vi "CC Script Parse Define.vi"(8 "error in (no error)":errorcluster, 9 "To String?":bool, 10 "Object in":T1, 11 "DefineObject Parameters":string="\"Object Name\" RA=12:32:25.123,DEC=45:22:33.234, muDEC=123.45, Epoch=12.345") -> (0 "error out":errorcluster, 1 "Name":string, 2 "Script":string, 3 "Object out":T1)   [LabVIEW 2024]
uses:
  typedefs/CC cluster Object.ctl
  typedefs/CC cluster sidereal rate.ctl
  typedefs/CC cluster RA and DEC.ctl
  typedefs/cc cluster muRA muDEC.ctl
  Telescope/CC cluster Telescope Offsets.ctl
  <vilib>/regexp/Match Regular Expression.xnode
panel:
  # "\"Object Name\" RA=HH:MM:SS.nnn,DEC=DEG:MM:SS.nnn, muDEC=nnn.nn, Epoch=nn.nnn"
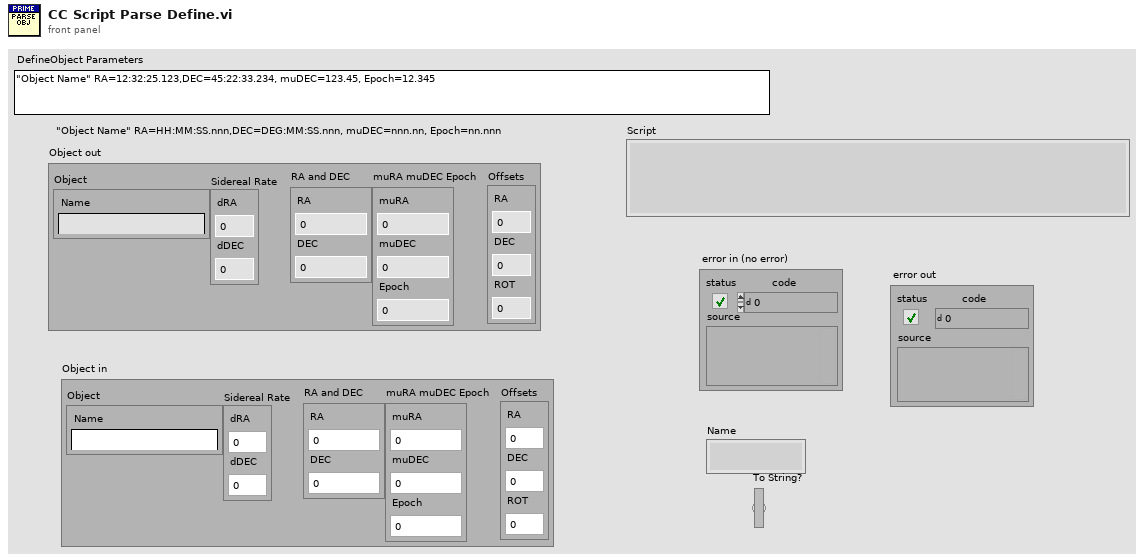
[diagram p1: front panel]
types:
  T1 = typedef "CC cluster Object.ctl" = cluster{"Object":cluster{"Name":string}, "Sidereal Rate":T2, "RA and DEC":T3, "muRA muDEC Epoch":T4, "Offsets":T5}
  T2 = typedef "CC cluster sidereal rate.ctl" = cluster{"dRA":dbl, "dDEC":dbl}
  T3 = typedef "CC cluster RA and DEC.ctl" = cluster{"RA":dbl, "DEC":dbl}
  T4 = typedef "cc cluster muRA muDEC.ctl" = cluster{"muRA":dbl, "muDEC":dbl, "Epoch":dbl}
  T5 = typedef "CC cluster Telescope Offsets.ctl" = cluster{"RA":dbl, "DEC":dbl, "ROT":dbl}
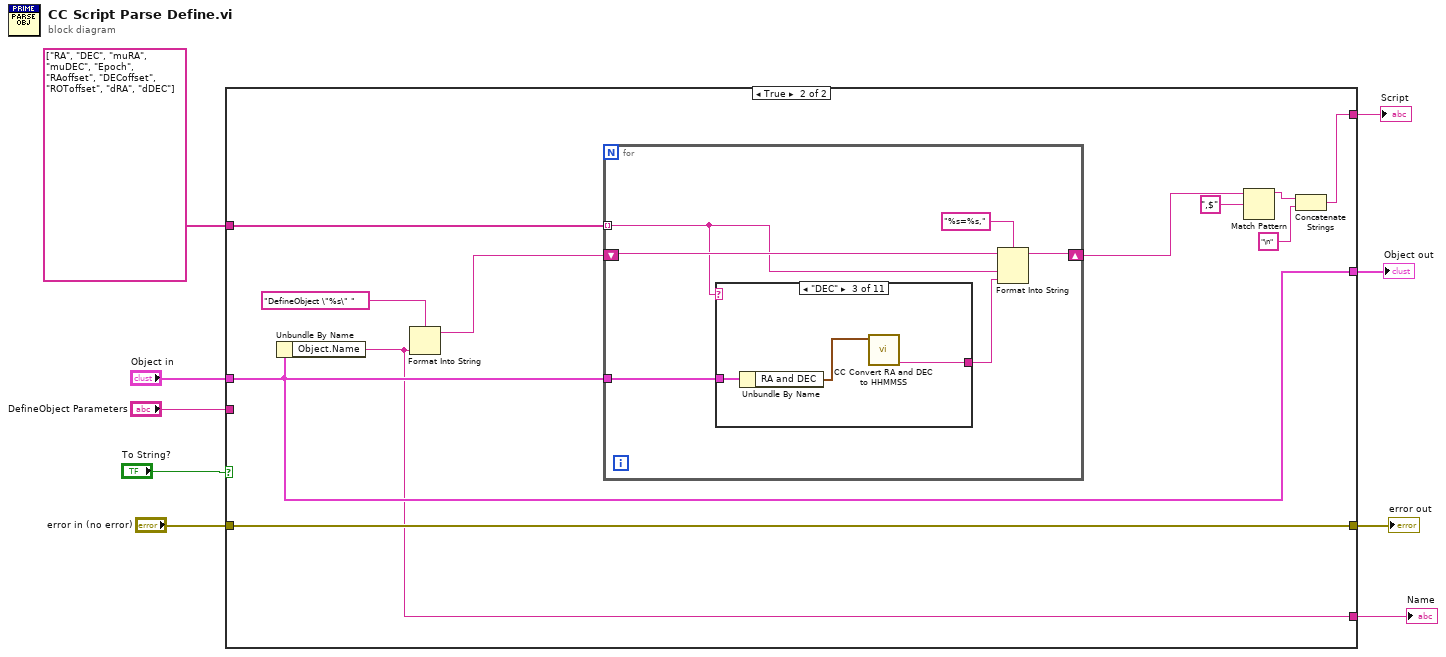
[diagram p0: block diagram]
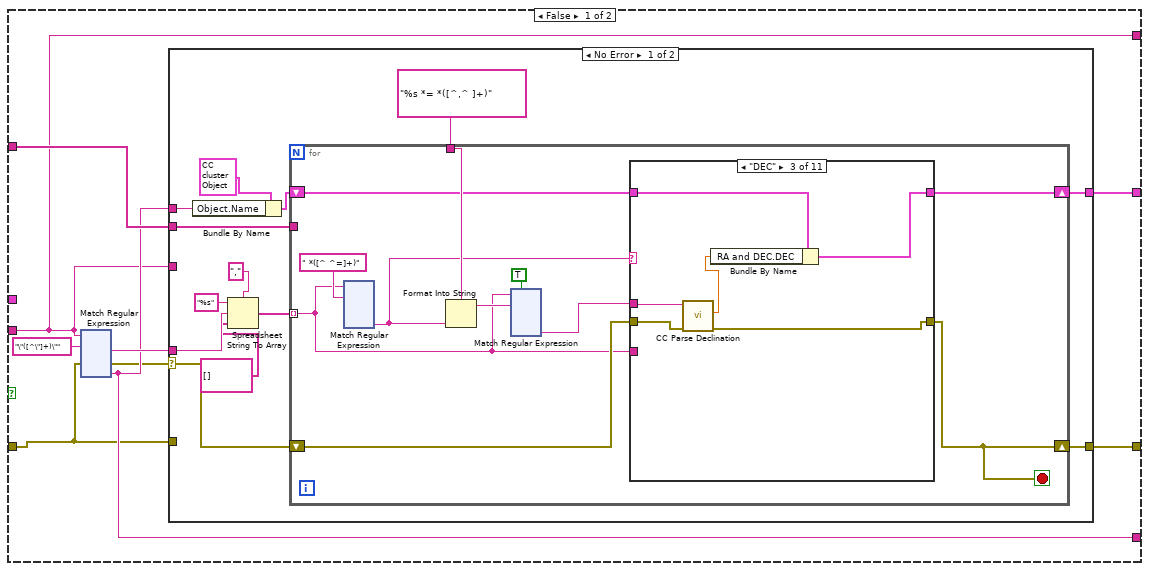
[diagram p2: hidden frame]
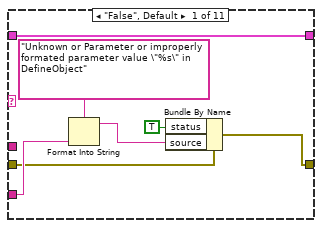
[diagram p3: hidden frame]
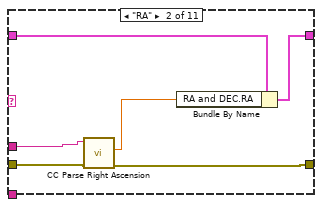
[diagram p4: hidden frame]
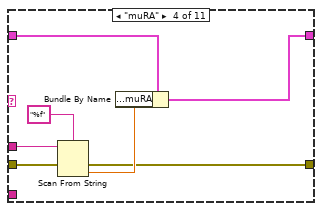
[diagram p5: hidden frame]
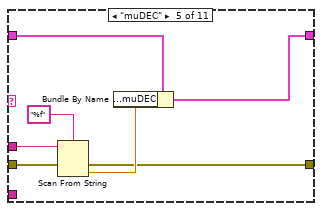
[diagram p6: hidden frame]
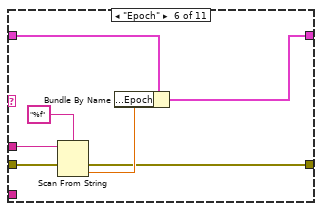
[diagram p7: hidden frame]
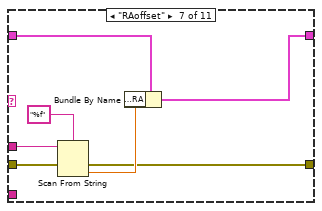
[diagram p8: hidden frame]
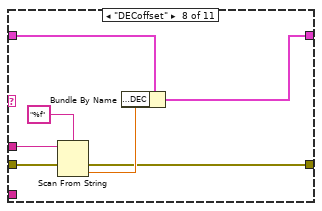
[diagram p9: hidden frame]
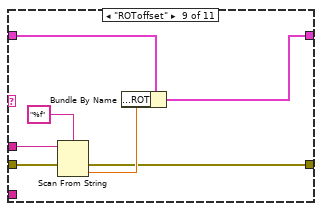
[diagram p10: hidden frame]
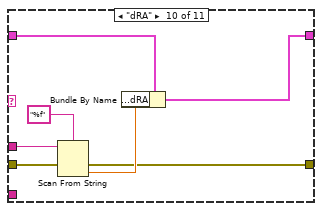
[diagram p11: hidden frame]
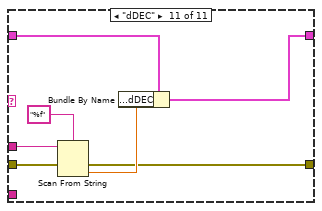
[diagram p12: hidden frame]
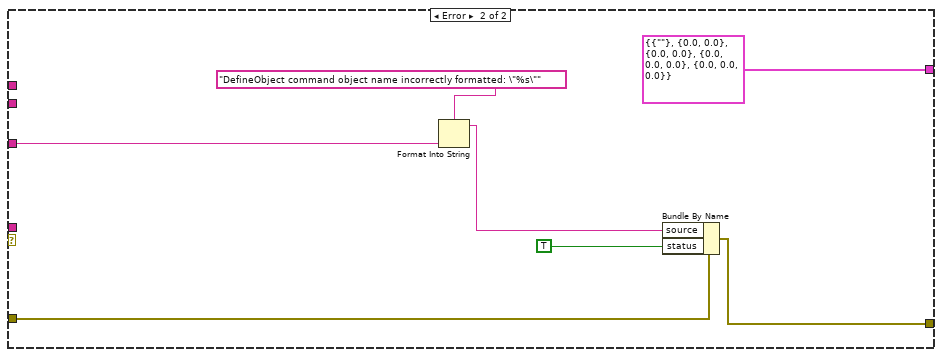
[diagram p13: hidden frame]
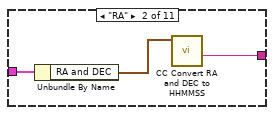
[diagram p15: hidden frame]
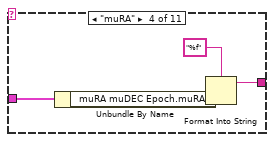
[diagram p16: hidden frame]
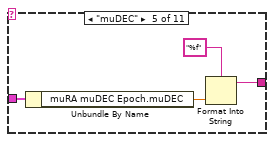
[diagram p17: hidden frame]
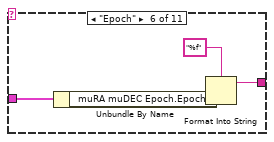
[diagram p18: hidden frame]
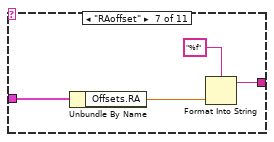
[diagram p19: hidden frame]
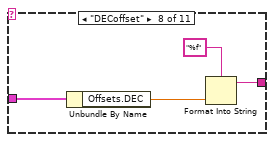
[diagram p20: hidden frame]
diagram:
  n1 = case shown="True" "To String?" {
    tunnel: "DefineObject Parameters" -> [w10 _]
    tunnel: string[] ["RA", "DEC", "muRA", "muDEC", "Epoch", "RAoffset", "DECoffset", "ROToffset", "dRA", "dDEC"] -> [w17 w491]
    tunnel: [w16 w483] -> w7
    tunnel: "error in (no error)" -> [w11 w489]
    tunnel: [w14 w489] -> w5
    tunnel: "Object in" -> [_ w483]
    tunnel: [w10 w484] -> w2
    tunnel: [w13 w482] -> w1
    frame False {
      n2 = xnode "Match Regular Expression"("input string"=w10, "regular expression"="\"([^\"]+)\"", "error in"=w11) -> ("after match"=w15:string, "error out"=w12:errorcluster, "submatch 1"=w13:string)  [unwired: 3 in, 3 out]
      n3 = case shown="No Error" w12 {
        selector: w12 -> [w24 _]
        tunnel: w17 -> [w31 _]
        tunnel: [w30 T1 {"Object"={"Name"=""}, "Sidereal Rate"={"dRA"=0.0, "dDEC"=0.0}, "RA and DEC"={"RA"=0.0, "DEC"=0.0}, "muRA muDEC Epoch"={"muRA"=0.0, "muDEC"=0.0, "Epoch"=0.0}, "Offsets"={"RA"=0.0, "DEC"=0.0, "ROT"=0.0}} ("Object")] -> w16
        tunnel: w15 -> [w23 _]
        tunnel: [w26 w357] -> w14
        tunnel: w13 -> [w25 _]
        tunnel: w11 -> [_ w362]
        tunnel: w10 -> [_ w359]
        frame No Error {
          n4 = Bundle By Name(cluster=T1 {"Object"={"Name"=""}, "Sidereal Rate"={"dRA"=0.0, "dDEC"=0.0}, "RA and DEC"={"RA"=0.0, "DEC"=0.0}, "muRA muDEC Epoch"={"muRA"=0.0, "muDEC"=0.0, "Epoch"=0.0}, "Offsets"={"RA"=0.0, "DEC"=0.0, "ROT"=0.0}} ("Object"), "Object.Name"=w25) -> (w27:T1)
          n5 = Spreadsheet String To Array(delimiter (Tab)=",", format string="%s", spreadsheet string=w23, array type (2D Dbl)=string[] []) -> (array=w19:string[])
          n6 = for {
            tunnel: "%s *= *([^,^ ]+)" ("regular expression") -> [w42]
            tunnel: w31 -> [_]
            shift-right: [w39] -> w30
            shift-left: w27 -> [w40]
            shift-right: [w32] -> w26
            shift-left: w24 -> [w37]
            tunnel: w19 -> [w33] mode=indexing
            stop <- w32 stop-if-true
            n7 = xnode "Match Regular Expression"("input string"=w33, "regular expression"=" *([^ ^=]+)" ("format string")) -> ("submatch 1"=w34:string)  [unwired: 4 in, 5 out]
            n8 = Format Into String(format string=w42, w34) -> (resulting string=w41:string)  [unwired: 2 in, 1 out]
            n9 = xnode "Match Regular Expression"("input string"=w33, "regular expression"=w41, "ignore case? (F)"=TRUE) -> ("submatch 1"=w38:string)  [unwired: 3 in, 5 out]
            n10 = case shown="\"DEC\"" w34 {
              tunnel: w40 -> [w168 w174 w180 w187 w194 w201 w208 w215 w222 w229 w236]
              tunnel: w38 -> [_ w170 w178 w185 w192 w199 w206 w213 w220 w227 w234]
              tunnel: [w168 w173 w179 w184 w191 w198 w205 w212 w219 w226 w233] -> w39
              tunnel: w37 -> [w162 w172 w177 w182 w189 w196 w203 w210 w217 w224 w231]
              tunnel: [w163 w171 w175 w181 w188 w195 w202 w209 w216 w223 w230] -> w32
              tunnel: w33 -> [w166 _ _ _ _ _ _ _ _ _ _]
              frame "False", Default {
                n11 = Format Into String(format string="Unknown or Parameter or improperly formated parameter value \"%s\" in DefineObject", w166) -> (resulting string=w165:string)  [unwired: 2 in, 1 out]
                n12 = Bundle By Name(cluster=w162, "status"=TRUE, "source"=w165) -> (w163:errorcluster)
              }
              frame "RA" {
                n13 = call "CC Parse Right Ascension.vi"("error in (no error)"=w172, "Right Ascension string"=w170) -> ("error out"=w171:errorcluster, "Angle"=w169:dbl)  [unwired: 7 in, 1 out]
                n14 = Bundle By Name(cluster=w174, "RA and DEC.RA"=w169) -> (w173:T1)
              }
              frame "DEC" {
                n15 = call "CC Parse Declination.vi"("error in (no error)"=w177, "Declination string"=w178) -> ("error out"=w175:errorcluster, "Angle"=w176:dbl)  [unwired: 7 in, 1 out]
                n16 = Bundle By Name(cluster=w180, "RA and DEC.DEC"=w176) -> (w179:T1)
              }
              frame "muRA" {
                n17 = Scan From String(format string="%f", input string=w185, error in=w182) -> (error out=w181:errorcluster, output 1=w183:dbl)  [unwired: 2 in, 2 out]
                n18 = Bundle By Name(cluster=w187, "muRA muDEC Epoch.muRA"=w183) -> (w184:T1)
              }
              frame "muDEC" {
                n19 = Scan From String(format string="%f", input string=w192, error in=w189) -> (error out=w188:errorcluster, output 1=w190:dbl)  [unwired: 2 in, 2 out]
                n20 = Bundle By Name(cluster=w194, "muRA muDEC Epoch.muDEC"=w190) -> (w191:T1)
              }
              frame "Epoch" {
                n21 = Scan From String(format string="%f", input string=w199, error in=w196) -> (error out=w195:errorcluster, output 1=w197:dbl)  [unwired: 2 in, 2 out]
                n22 = Bundle By Name(cluster=w201, "muRA muDEC Epoch.Epoch"=w197) -> (w198:T1)
              }
              frame "RAoffset" {
                n23 = Scan From String(format string="%f", input string=w206, error in=w203) -> (error out=w202:errorcluster, output 1=w204:dbl)  [unwired: 2 in, 2 out]
                n24 = Bundle By Name(cluster=w208, "Offsets.RA"=w204) -> (w205:T1)
              }
              frame "DECoffset" {
                n25 = Scan From String(format string="%f", input string=w213, error in=w210) -> (error out=w209:errorcluster, output 1=w211:dbl)  [unwired: 2 in, 2 out]
                n26 = Bundle By Name(cluster=w215, "Offsets.DEC"=w211) -> (w212:T1)
              }
              frame "ROToffset" {
                n27 = Scan From String(format string="%f", input string=w220, error in=w217) -> (error out=w216:errorcluster, output 1=w218:dbl)  [unwired: 2 in, 2 out]
                n28 = Bundle By Name(cluster=w222, "Offsets.ROT"=w218) -> (w219:T1)
              }
              frame "dRA" {
                n29 = Scan From String(format string="%f", input string=w227, error in=w224) -> (error out=w223:errorcluster, output 1=w225:dbl)  [unwired: 2 in, 2 out]
                n30 = Bundle By Name(cluster=w229, "Sidereal Rate.dRA"=w225) -> (w226:T1)
              }
              frame "dDEC" {
                n31 = Scan From String(format string="%f", input string=w234, error in=w231) -> (error out=w230:errorcluster, output 1=w232:dbl)  [unwired: 2 in, 2 out]
                n32 = Bundle By Name(cluster=w236, "Sidereal Rate.dDEC"=w232) -> (w233:T1)
              }
            }
          }
        }
        frame Error {
          n33 = Format Into String(format string="DefineObject command object name incorrectly formatted: \"%s\"", w359) -> (resulting string=w358:string)  [unwired: 2 in, 1 out]
          n34 = Bundle By Name(cluster=w362, "source"=w358, "status"=TRUE) -> (w357:errorcluster)
        }
      }
    }
    frame True {
      n35 = Unbundle By Name(w483) -> ("Object.Name"=w482:string)
      n36 = Format Into String(format string="DefineObject \"%s\" ", w482) -> (resulting string=w490:string)  [unwired: 2 in, 1 out]
      n37 = for {
        tunnel: w491 -> [w495] mode=indexing
        shift-right: [w493] -> w488
        shift-left: w490 -> [w497]
        tunnel: w483 -> [w498]
        n38 = case shown="\"DEC\"" w495 {
          tunnel: w498 -> [_ w501 w504 w508 w512 w516 w520 w524 w528 w532 w536]
          tunnel: [_ w499 w502 w505 w509 w513 w517 w521 w525 w529 w533] -> w494
          frame "False", Default {
          }
          frame "RA" {
            n39 = Unbundle By Name(w501) -> ("RA and DEC"=w500:T3)
            n40 = call "CC Convert RA and DEC to HHMMSS.vi"("RA and DEC"=w500) -> ("RA String"=w499:string)  [unwired: 9 in, 1 out]
          }
          frame "DEC" {
            n41 = Unbundle By Name(w504) -> ("RA and DEC"=w503:T3)
            n42 = call "CC Convert RA and DEC to HHMMSS.vi"("RA and DEC"=w503) -> ("DEC String"=w502:string)  [unwired: 9 in, 1 out]
          }
          frame "muRA" {
            n43 = Unbundle By Name(w508) -> ("muRA muDEC Epoch.muRA"=w506:dbl)
            n44 = Format Into String(format string="%f", w506) -> (resulting string=w505:string)  [unwired: 2 in, 1 out]
          }
          frame "muDEC" {
            n45 = Unbundle By Name(w512) -> ("muRA muDEC Epoch.muDEC"=w510:dbl)
            n46 = Format Into String(format string="%f", w510) -> (resulting string=w509:string)  [unwired: 2 in, 1 out]
          }
          frame "Epoch" {
            n47 = Unbundle By Name(w516) -> ("muRA muDEC Epoch.Epoch"=w514:dbl)
            n48 = Format Into String(format string="%f", w514) -> (resulting string=w513:string)  [unwired: 2 in, 1 out]
          }
          frame "RAoffset" {
            n49 = Unbundle By Name(w520) -> ("Offsets.RA"=w518:dbl)
            n50 = Format Into String(format string="%f", w518) -> (resulting string=w517:string)  [unwired: 2 in, 1 out]
          }
          frame "DECoffset" {
            n51 = Unbundle By Name(w524) -> ("Offsets.DEC"=w522:dbl)
            n52 = Format Into String(format string="%f", w522) -> (resulting string=w521:string)  [unwired: 2 in, 1 out]
          }
          frame "ROToffset" {
            n53 = Unbundle By Name(w528) -> ("Offsets.ROT"=w526:dbl)
            n54 = Format Into String(format string="%f", w526) -> (resulting string=w525:string)  [unwired: 2 in, 1 out]
          }
          frame "dRA" {
            n55 = Unbundle By Name(w532) -> ("Sidereal Rate.dRA"=w530:dbl)
            n56 = Format Into String(format string="%f", w530) -> (resulting string=w529:string)  [unwired: 2 in, 1 out]
          }
          frame "dDEC" {
            n57 = Unbundle By Name(w536) -> ("Sidereal Rate.dDEC"=w534:dbl)
            n58 = Format Into String(format string="%f", w534) -> (resulting string=w533:string)  [unwired: 2 in, 1 out]
          }
        }
        n59 = Format Into String(format string="%s=%s,", initial string=w497, w495, w494) -> (resulting string=w493:string)  [unwired: 1 in, 1 out]
      }
      n60 = Match Pattern(string=w488, regular expression=",$") -> (before substring=w486:string)  [unwired: 1 in, 3 out]
      n61 = Concatenate Strings(w486, "\n" ("string")) -> (w484:string)
    }
  }
  "error out" <- w5
  "Object out" <- w7
  "Script" <- w2
  "Name" <- w1
